vi "PH_AxisGUI_NF.get i attribute.vi"(0 "i ref in":refnum<vi>, 5 "error in (no error)":errorcluster) -> (14 "i ref out":refnum<vi>, 16 "i attribute":T1={"GUI Refs"={"Delete"=refnum, "Slide 0"=refnum, "Slide 1"=refnum, "Slide 2"=refnum, "Instance Status"=refnum, "Position"=refnum, "Reset"=refnum, "Goal"=refnum, "Go"=refnum}, "Instance"="N/A", "Name Axis 0"="N/A", "Name Axis 1"="N/A", "Name Axis 2"="N/A", "System"="N/A", "Driver Type"=enum."not defined", "Offset"=0, "Goal"=0}, 19 "error out":errorcluster)   [LabVIEW 2014, in "PH_AxisGUI_NF.lvlib"]
doc: "Gets the i attribute data of an object.\n\nLicense Agreement for this software:\n\nCopyright (C)\nGesellschaft für Schwerionenforschung, GSI\nPlanckstr. 1\n64291 Darmstadt\nGermany\n\nContact: D.Beck@gsi.de \n\nThis program is free software; you can redistribute it and/or modify it under the terms of the GNU General Public License as published by the Free Software Foundation; either version 2 of the license, or (at your option) any later version.\n\nThis program is distributed in the hope that it will be useful, but WITHOUT ANY WARRANTY; without even the implied warranty of MERCHANTABILITY or FITNESS FOR A PARTICULAR PURPOSE. See the GNU General License for more details (http://www.gnu.org).\n\nGesellschaft für Schwerionenforschung, GSI\nPlanckstr. 1, 64291 Darmstadt, Germany\nFor all questions and ideas contact: M.Richter@gsi.de, H.Brand@gsi.de or D.Beck@gsi.de.\nLast update: 17-JUN-2004"
uses:
  PH_AxisGUI_NF.lvlib
  PH_AxisGUI_NF.i attribute.ctl
  CSMotion/NF87XX/NF87XX.driver Type.ctl
  CSMotion/NF87XX/NF87XX.lvlib
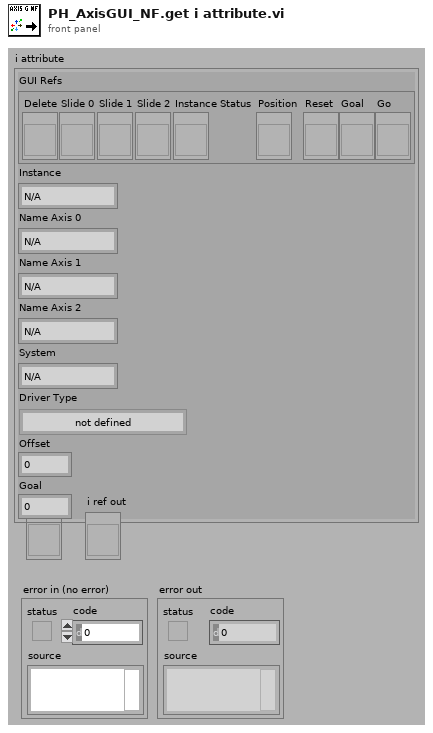
[diagram p1: front panel]
types:
  T1 = typedef "PH_AxisGUI_NF.lvlib/PH_AxisGUI_NF.i attribute.ctl" = cluster{"GUI Refs":cluster{"Delete":refnum<vi>, "Slide 0":refnum<vi>, "Slide 1":refnum<vi>, "Slide 2":refnum<vi>, "Instance Status":refnum<vi>, "Position":refnum<vi>, "Reset":refnum<vi>, "Goal":refnum<vi>, "Go":refnum<vi>}, "Instance":string, "Name Axis 0":string, "Name Axis 1":string, "Name Axis 2":string, "System":string, "Driver Type":T2, "Offset":i32, "Goal":i32}
  T2 = typedef "NF87XX.lvlib/NF87XX.driver Type.ctl" = enum16{"not defined", "3-ch open loop drv", "1-ch closed loop drv"}
  T3 = enum16{"SetAttribute", "GetAttribute", "CreateAttribute", "DestroyAttribute", "DestroyAllAtributes"}
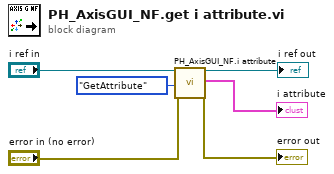
[diagram p0: block diagram]
diagram:
  n1 = call "PH_AxisGUI_NF.i attribute.vi"("VI Refnum"="i ref in", "Action"=T3."GetAttribute", "error in (no error)"="error in (no error)") -> ("VI Refnum out"=→"i ref out":refnum<vi>, "CLASS.i attribute out"=→"i attribute":T1, "error out"=→"error out":errorcluster)  [unwired: 14 in]
